vi "Is Form Submission.vi"(8 "error in (no error)":errorcluster, 11 "Request in":refnum<class "Request.lvclass">) -> (0 "error out":errorcluster, 2 "Is Form Submission?":bool, 3 "Request out":refnum<class "Request.lvclass">)   [LabVIEW 2020, in "HTTP Utils.lvlib" / "Request.lvclass"]
uses:
  Request.lvclass
  Request.lvclass/Request.ctl
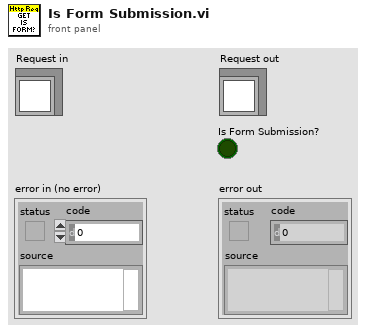
[diagram p1: front panel]
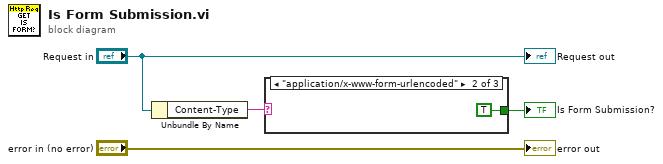
[diagram p0: block diagram]
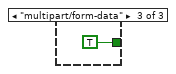
[diagram p3: hidden frame]
diagram:
  n1 = Unbundle By Name("Request in") -> ("Content-Type"=w2:string)
  n2 = case shown="\"application/x-www-form-urlencoded\"" w2 {
    tunnel: [_ TRUE TRUE] -> w1
    frame Default {
    }
    frame "application/x-www-form-urlencoded" {
    }
    frame "multipart/form-data" {
    }
  }
  "Is Form Submission?" <- w1
  "error out" <- "error in (no error)"
  "Request out" <- "Request in"
